vi "PRM1Z8_setPower.vi"(4 "zero angle":dbl, 6 "max power":dbl=6000.0, 7 "Target Power":dbl, 8 "error in (no error)":errorcluster, 11 "reference":refnum<k24>) -> (0 "error out":errorcluster, 3 "reference out":refnum<k24>)   [LabVIEW 2023, in "Thorlabs Polarizer.lvlib"]
uses:
  C:/FlashGordon/Development/dll/ThorLabs.MotionControl.KCube.DCServoCLI.dll
  dll/ThorLabs.MotionControl.KCube.DCServoCLI.dll
  Thorlabs Polarizer.lvlib
panel:
  out "output angle":dbl
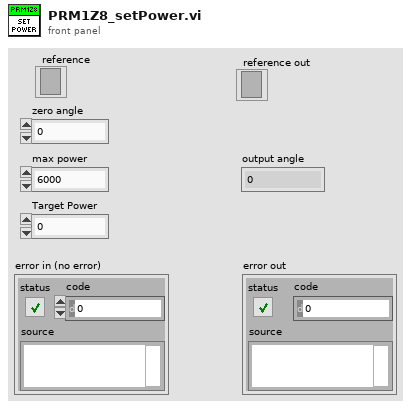
[diagram p1: front panel]
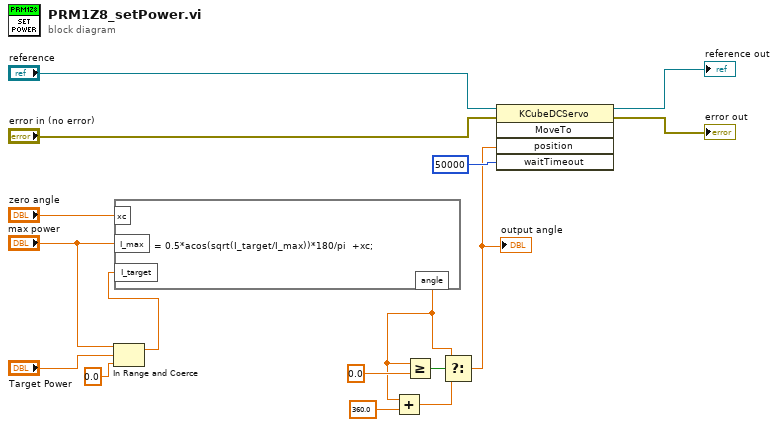
[diagram p0: block diagram]
diagram:
  n1 = In Range and Coerce(upper limit="max power", x="Target Power", lower limit=0.0) -> (coerced(x)=w5:dbl)  [unwired: 1 out]
  n2 = formula code="angle = 0.5*acos(sqrt(I_target/I_max))*180/pi  +xc;"("I_target"=w5, "I_max"="max power", "xc"="zero angle") -> ("angle"=w9:dbl)
  n3 = Add(x=w9, y=360.0) -> (x+y=w12:dbl)
  n4 = Greater Or Equal?(x=w9, y=0.0) -> (x >= y?=w8:bool)
  n5 = Select(t=w9, s=w8, f=w12) -> (s? t:f=w13:dbl)
  "output angle" <- w13
  n6 = invoke class="KCubeDCServo" method="MoveTo"(reference="reference", error in="error in (no error)", "position"=w13, "waitTimeout"=50000) -> (reference out=→"reference out":refnum<k24>, error out=→"error out":errorcluster)  [unwired: 1 in, 3 out]
